vi "Write I32.vi"(8 "error in (no error)":errorcluster, 10 "I32":i32, 11 "Section 2a in":refnum<class "Section 2a.lvclass">) -> (0 "error out":errorcluster, 3 "Section 2a out":refnum<class "Section 2a.lvclass">)   [LabVIEW 2013, in "LVOOP Introduction.lvlib" / "Section 2a.lvclass"]
uses:
  Section 2a.lvclass
  Section 2a.lvclass/Section 2a.ctl
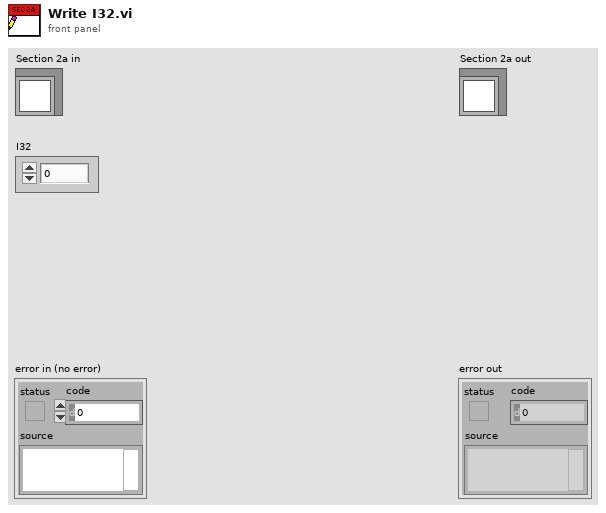
[diagram p1: front panel]
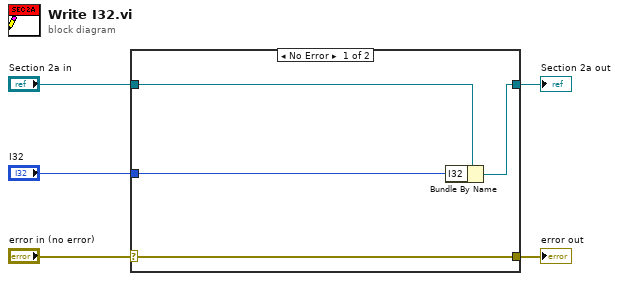
[diagram p0: block diagram]
diagram:
  n1 = case shown="No Error" "error in (no error)" {
    selector: "error in (no error)" -> [w9 w10]
    tunnel: [w9 w10] -> w4
    tunnel: [w7 w11] -> w2
    tunnel: "Section 2a in" -> [w8 w11]
    tunnel: "I32" -> [w6 _]
    frame No Error {
      n2 = Bundle By Name(cluster=w8, "I32"=w6) -> (w7:refnum<class "Section 2a.lvclass">)
    }
    frame Error {
    }
  }
  "error out" <- w4
  "Section 2a out" <- w2
